vi "REV2_Bulk_Stat.vi"(6 "Stat_to_Read":T1[](array[typedef]) items=["Torque Enable", "Homing Complete", "Goal Id", "Goal Iq", "Goal Velo", "Goal Posi", "Present Id", "Present Iq", "Present Velo", "Present Posi", "Bus Voltage", "Temperature Winding", "Temperature MOSFET", "Temperature IC", "Error Status", "Iq_Temps"], 7 "IDs":u8[](array[numeric]), 8 "error in (no error)":errorcluster, 9 "Data_to_Write":dbl[][](array[numeric]), 10 "Stat_to_Write":T1[](array[typedef]) items=["Torque Enable", "Homing Complete", "Goal Id", "Goal Iq", "Goal Velo", "Goal Posi", "Present Id", "Present Iq", "Present Velo", "Present Posi", "Bus Voltage", "Temperature Winding", "Temperature MOSFET", "Temperature IC", "Error Status", "Iq_Temps"], 11 "VISA Refnum in":refnum<visa-resource-name>) -> (0 "error out":errorcluster, 2 "Data_2D":dbl[][](array[numeric]), 3 "VISA Refnum out":refnum<visa-resource-name>)   [LabVIEW 2016, in "REV_2.lvlib"]
uses:
  REV_2.lvlib
  REV2_Instructions.ctl
  REV2_Stat_Addr.ctl
panel:
  out "ERROR":u8
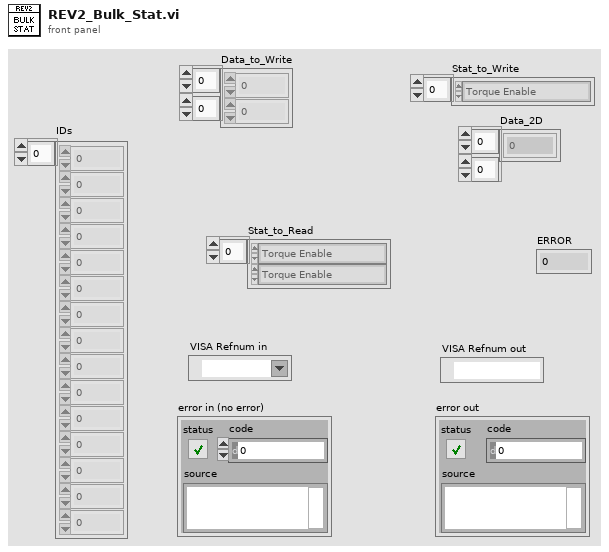
[diagram p1: front panel]
types:
  T1 = typedef "REV_2.lvlib/REV2_Stat_Addr.ctl" = u8
  T2 = enum16{"big-endian, network order", "native, host order", "little-endian"}
  T3 = typedef "REV_2.lvlib/REV2_Instructions.ctl" = u8
  T4 = cluster{"ID":u8, "ERROR":u8, "ChechSumError?":bool, "Data":string}
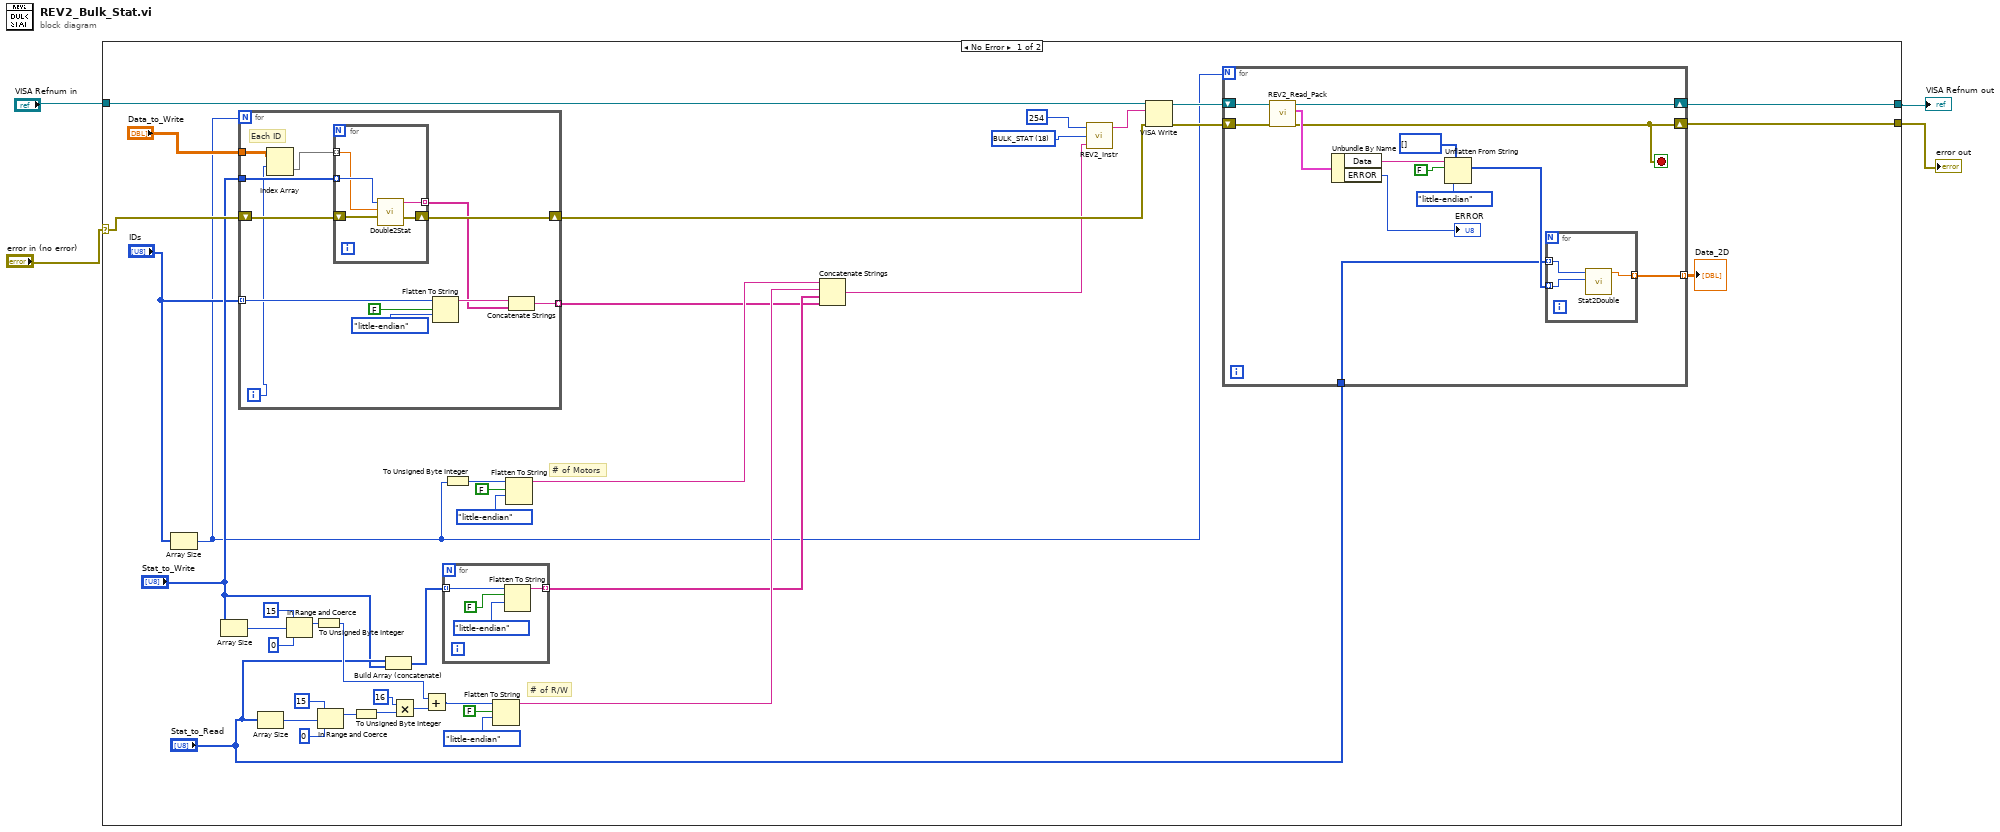
[diagram p0: block diagram]
diagram:
  n1 = case shown="No Error" "error in (no error)" {
    selector: "error in (no error)" -> [w42 w83]
    tunnel: [w38 w82] -> w4
    tunnel: [w37 w83] -> w3
    tunnel: "VISA Refnum in" -> [w44 w82]
    frame No Error {
      w8 = T3 18 items=["PING"=1, "READ_STAT"=2, "WRITE_STAT"=3, "READ_CONFIG"=4, "WRITE_CONFIG"=5, "SAVE_CONFIG"=6, "BULK_STAT"=18] ("Instruction")
      # "# of R/W"
      # "# of Motors"
      n2 = Array Size(array="IDs") -> (size(s)=w7:i32)
      n3 = Array Size(array="Stat_to_Write") -> (size(s)=w33:i32)
      n4 = for {
        N: w7 -> [_]
        tunnel: "Stat_to_Write" -> [w70]
        shift-right: [w72] -> w43
        shift-left: w42 -> [w71]
        tunnel: "Data_to_Write" -> [w63]
        tunnel: "IDs" -> [w67] mode=indexing
        tunnel: [w64] -> w10 mode=indexing
        i -> [w62]
        # "Each ID"
        n5 = Index Array(array=w63, index (row)=w62) -> (element=w61:dbl[])  [unwired: 1 in]
        n6 = for {
          tunnel: w70 -> [w77] mode=indexing
          shift-right: [w75] -> w72
          shift-left: w71 -> [w76]
          tunnel: w61 -> [w74] mode=indexing
          tunnel: [w73] -> w65 mode=indexing
          n7 = call "Double2Stat.vi"("error in (no error)"=w76, "Data"=w74, "Stat Address"=w77) -> ("error out"=w75:errorcluster, "data string"=w73:string)  [unwired: 7 in]
        }
        n8 = Flatten To String(anything=w67, prepend array or string size? (T)=FALSE, byte order (0:big-endian, network order)=T2."little-endian") -> (data string=w66:string)  [unwired: 1 in, 2 out]
        n9 = Concatenate Strings(w66, w65) -> (w64:string)
      }
      n10 = Array Size(array="Stat_to_Read") -> (size(s)=w26:i32)
      n11 = In Range and Coerce(upper limit=15, x=w33, lower limit=0) -> (coerced(x)=w32:i32)  [unwired: 1 out]
      n12 = To Unsigned Byte Integer(number=w32) -> (unsigned 8bit integer=w17:u8)
      n13 = In Range and Coerce(upper limit=15, x=w26, lower limit=0) -> (coerced(x)=w27:i32)  [unwired: 1 out]
      n14 = To Unsigned Byte Integer(number=w27) -> (unsigned 8bit integer=w25:u8)
      n15 = Build Array (concatenate)("Stat_to_Read", "Stat_to_Write") -> (w14:T1[])
      n16 = Multiply(x=u8 16, y=w25) -> (x*y=w23:u8)
      n17 = Add(x=w17, y=w23) -> (x+y=w20:u8)
      n18 = for {
        tunnel: w14 -> [w79] mode=indexing
        tunnel: [w78] -> w13 mode=indexing
        n19 = Flatten To String(anything=w79, prepend array or string size? (T)=FALSE, byte order (0:big-endian, network order)=T2."little-endian") -> (data string=w78:string)  [unwired: 1 in, 2 out]
      }
      n20 = To Unsigned Byte Integer(number=w7) -> (unsigned 8bit integer=w34:u8)
      n21 = Flatten To String(anything=w20, prepend array or string size? (T)=FALSE, byte order (0:big-endian, network order)=T2."little-endian") -> (data string=w18:string)  [unwired: 1 in, 2 out]
      n22 = Flatten To String(anything=w34, prepend array or string size? (T)=FALSE, byte order (0:big-endian, network order)=T2."little-endian") -> (data string=w19:string)  [unwired: 1 in, 2 out]
      n23 = Concatenate Strings(w19, w18, w13, w10) -> (w9:string)
      n24 = call "REV2_Instr.vi"("Parameter"=w9, "Instruction"=w8, "ID"=u8 254) -> ("Output"=w5:string)  [unwired: 2 in]
      n25 = VISA Write(VISA resource name=w44, write buffer=w5, error in (no error)=w43) -> (VISA resource name out=w39:refnum<visa-resource-name>, error out=w40:errorcluster)  [unwired: 1 out]
      n26 = for {
        N: w7 -> [_]
        shift-right: [w47] -> w37
        shift-left: w40 -> [w50]
        shift-right: [w48] -> w38
        shift-left: w39 -> [w49]
        tunnel: [w46] -> w6 mode=indexing
        tunnel: "Stat_to_Read" -> [w45]
        stop <- w47 stop-if-true
        n27 = call "REV2_Read_Pack.vi"("error in (no error)"=w50, "VISA Refnum in"=w49) -> ("error out"=w47:errorcluster, "output cluster"=w56:T4, "VISA Refnum out"=w48:refnum<visa-resource-name>)  [unwired: 7 in]
        n28 = Unbundle By Name(w56) -> ("Data"=w51:string, "ERROR"=→"ERROR":u8)
        n29 = Unflatten From String(type=u32[] [], binary string=w51, data includes array or string size? (T)=FALSE, byte order (0:big-endian, network order)=T2."little-endian") -> (value=w57:u32[])  [unwired: 1 in, 2 out]
        n30 = for {
          tunnel: w45 -> [w60] mode=indexing
          tunnel: w57 -> [w59] mode=indexing
          tunnel: [w58] -> w46 mode=indexing
          n31 = call "Stat2Double.vi"("Numeric in"=w59, "Stat Address"=w60) -> ("Numeric out"=w58:dbl)  [unwired: 9 in]
        }
      }
      "Data_2D" <- w6
    }
    frame Error {
    }
  }
  "VISA Refnum out" <- w4
  "error out" <- w3
